vi "Set Frequency and Phase.vi"(5 "CS Channel":u8, 6 "Ref Clock Freq (125MHz)":dbl=125000000.0 format="%#_6p", 7 "SPI Channel (0)":u8, 8 "Error In":errorcluster, 9 "Phase Offset (5-bit)":u8, 10 "Frequency":u32, 11 "LINX Resource":T1) -> (0 "Error Out":errorcluster, 3 "LINX Resource":T1)   [LabVIEW 2011, in "LVH-LINX.lvlib" / "AD9850.lvlib"]
uses:
  AD9850.lvlib
  Private/Type Defs/LINX Ref.ctl
  Private/Type Defs/Platform.ctl
  Private/Type Defs/Interface.ctl
  Private/Device/Type Defs/LINX Device Config.ctl
  Private/Device/Type Defs/TCP Config.ctl
  Private/Device/Type Defs/Channels.ctl
  Peripherals/SPI/SPI CS Config.ctl
  Private/Type Defs/Peripherals/SPI/SPI CS Logic Level.ctl
  Peripherals/SPI/SPI Write Read 1 Frame.vi
  LVH-LINX.lvlib
  Private/Device/Device.lvlib
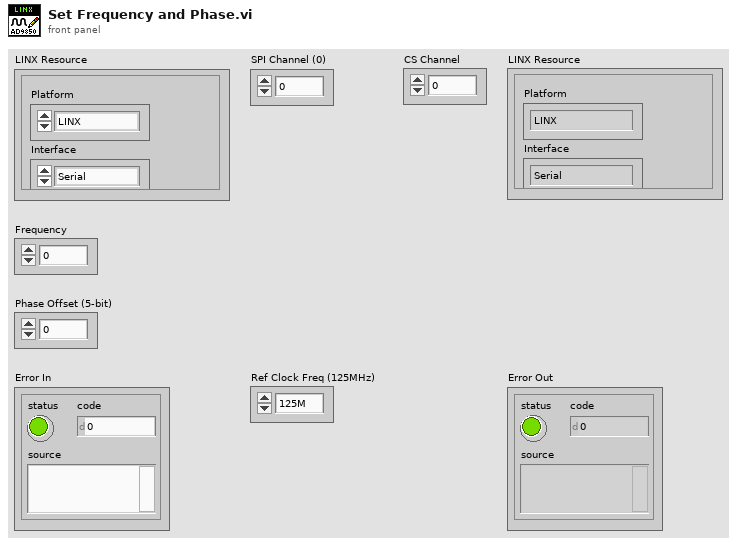
[diagram p1: front panel]
types:
  T1 = typedef "LVH-LINX.lvlib/LINX Ref.ctl" = cluster{"Platform":T2, "Interface":T3, "LINX Device Config":T4}
  T2 = typedef "LVH-LINX.lvlib/Platform.ctl" = enum16{"LINX", "myRIO"}
  T3 = typedef "LVH-LINX.lvlib/Interface.ctl" = enum16{"Serial", "TCP"}
  T4 = typedef "LVH-LINX.lvlib/Device.lvlib/LINX Device Config.ctl" = cluster{"Interface":T3, "COM Port":refnum<visa-resource-name>, "TCP Configuration":T5, "Device Family":u8, "Device ID":u8, "Device Name":string, "TCP Ref":refnum<k5>, "Channels":T6}
  T5 = typedef "LVH-LINX.lvlib/Device.lvlib/TCP Config.ctl" = cluster{"IP Address":string, "Port":u16}
  T6 = typedef "LVH-LINX.lvlib/Channels.ctl" = cluster{"DI":u8[], "DO":u8[], "AI":u8[], "AO":u8[], "PWM":u8[], "QE":u8[], "UART":u8[], "I2C 2":u8[], "SPI":u8[], "CAN":u8[], "Servo":u8[], "AI Ref (V)":dbl, "AO Ref (V)":dbl, "AO Resolution (Bits)":u8}
  T7 = typedef "LVH-LINX.lvlib/SPI CS Config.ctl" = cluster{"CS Channel":u8, "CS Logic Level":T8}
  T8 = typedef "LVH-LINX.lvlib/SPI CS Logic Level.ctl" = enum8{"Active Low", "Active High"}
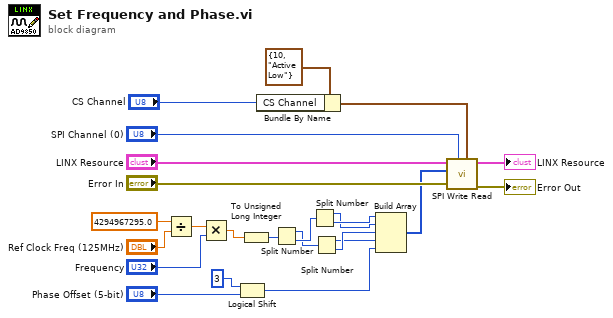
[diagram p0: block diagram]
diagram:
  n1 = Divide(x=4294967295.0, y="Ref Clock Freq (125MHz)") -> (x/y=w18:dbl)
  n2 = Multiply(x=w18, y="Frequency") -> (x*y=w12:dbl)
  n3 = Logical Shift(y=i8 3, x="Phase Offset (5-bit)") -> (x << y=w10:u8)
  n4 = To Unsigned Long Integer(number=w12) -> (unsigned 32bit integer=w11:u32)
  n5 = Bundle By Name(cluster=T7 {"CS Channel"=10, "CS Logic Level"=enum."Active Low"} ("CS Configuration"), "CS Channel"="CS Channel") -> (w1:T7)
  n6 = Split Number(x=w11) -> (hi(x)=w19:u16, lo(x)=w20:u16)
  n7 = Split Number(x=w20) -> (hi(x)=w23:u8, lo(x)=w24:u8)
  n8 = Split Number(x=w19) -> (hi(x)=w21:u8, lo(x)=w22:u8)
  n9 = Build Array(w24, w23, w22, w21, w10) -> (w5:u8[])
  n10 = call-poly "SPI Write Read.vi"("CS Configuration"=w1, "SPI Channel (0)"="SPI Channel (0)", "Error In"="Error In", "Data"=w5, "LINX Resource"="LINX Resource") -> ("Error Out"=→"Error Out":errorcluster, "LINX Resource"=→"LINX Resource":T1)  [unwired: 4 in, 1 out]
